vi "Anritsu VNA Set Measurement.vi"(4 "Trace":i8=1 min=1 max=99 step=1, 5 "Parameter":T2={"Stimulus Port"=1, "Response Port"=1} {"Stimulus Port" min=1 step=1; "Response Port" min=1 step=1}, 6 "Channel":i8=1 min=1 max=99 step=1, 7 "Anritsu VNA":T1, 8 "error in (no error)":errorcluster, 11 "VISA Resource Name":refnum<visa-resource-name>) -> (0 "error out":errorcluster, 3 "dup VISA Resource Name":refnum<visa-resource-name>)   [LabVIEW 2011]
doc: "This VI for the HP8753B Network Analyzer sets the measurement."
uses:
  tests/S Parameter/TypeDefs/SP Parameter.ctl
  TypeDefs/Anritsu VNA Instrument Info.ctl
  TypeDefs/Anritsu VNA MS2024A and MS2026A Measurement.ctl
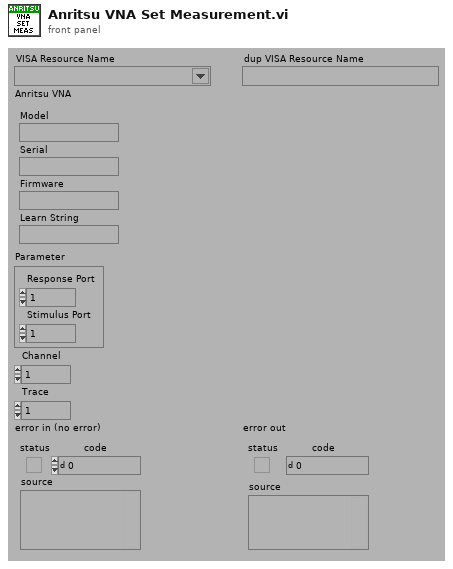
[diagram p1: front panel]
types:
  T1 = typedef "Anritsu VNA Instrument Info.ctl" = cluster{"Model":string, "Serial":string, "Firmware":string, "Learn String":string}
  T2 = typedef "SP Parameter.ctl" = cluster{"Stimulus Port":i8, "Response Port":i8}
  T3 = typedef "Anritsu VNA Model.ctl" = enum16{"Not Supported", "37XXXX", "MS20XXX", "MS462XX", "MS464XX"}
  T4 = typedef "Anritsu VNA MS2024A and MS2026A Measurement.ctl" = enum32{"S11 - Group Delay", "S11 - Log Mag Fault Location", "S11 - Log Mag", "S11 - Phase", "S11 - Smith", "S11 - VSWR Fault Location", "S11 - VSWR", "S21 - Group Delay", "S21 - Log Mag", "S21 - Phase"}
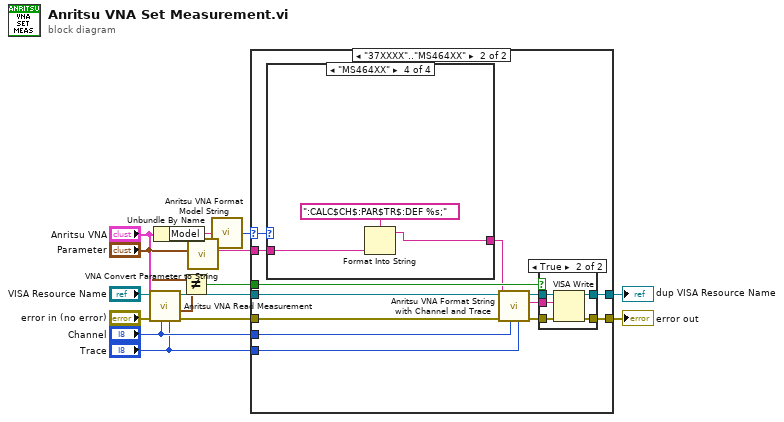
[diagram p0: block diagram]
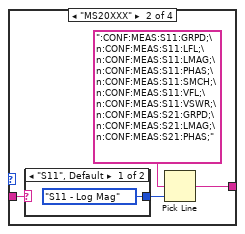
[diagram p5: hidden frame]
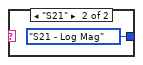
[diagram p6: hidden frame]
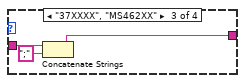
[diagram p7: hidden frame]
diagram:
  n1 = call "Anritsu VNA Read Measurement.vi"("Trace"="Trace", "Channel"="Channel", "Anritsu VNA"="Anritsu VNA", "error in (no error)"="error in (no error)", "VISA Resource Name"="VISA Resource Name") -> ("error out"=w10:errorcluster, "Parameter"=w3:T2, "dup VISA Resource Name"=w9:refnum<visa-resource-name>)  [unwired: 1 in, 3 out]
  n2 = Unbundle By Name("Anritsu VNA") -> ("Model"=w5:string)
  n3 = Not Equal?(x="Parameter", y=w3) -> (x != y?=w7:bool)
  n4 = call "VNA Convert Parameter to String.vi"("Parameter"="Parameter") -> ("Parameter String"=w13:string)  [unwired: 10 out]
  n5 = call "Anritsu VNA Format Model String.vi"("Model"=w5) -> ("Model"=w4:T3)
  n6 = case shown="\"37XXXX\"..\"MS464XX\"" w4 {
    selector: w4 -> [_ w22]
    tunnel: [w17 w28] -> w15
    tunnel: [w16 w27] -> w14
    tunnel: w13 -> [_ w26]
    tunnel: w10 -> [w16 w25]
    tunnel: w9 -> [w17 w24]
    tunnel: w7 -> [_ w23]
    tunnel: "Trace" -> [_ w19]
    tunnel: "Channel" -> [_ w18]
    frame "Not Supported" {
    }
    frame "37XXXX".."MS464XX" {
      n7 = case shown="\"MS464XX\"" w22 {
        tunnel: [_ w38 w44 w45] -> w20
        tunnel: w26 -> [_ w37 w42 w46]
        frame "Not Supported" {
        }
        frame "MS20XXX" {
          n8 = case shown="\"S11\", Default" w37 {
            tunnel: [Anritsu_VNA_MS2024A_and_MS2026A_Measurement."S11 - Log Mag" ("Measurement (S11 - Log Mag)") Anritsu_VNA_MS2024A_and_MS2026A_Measurement."S21 - Log Mag" ("Measurement (S11 - Log Mag)")] -> w36
            frame "S11", Default {
            }
            frame "S21" {
            }
          }
          n9 = Pick Line(multi-line string=":CONF:MEAS:S11:GRPD;\n:CONF:MEAS:S11:LFL;\n:CONF:MEAS:S11:LMAG;\n:CONF:MEAS:S11:PHAS;\n:CONF:MEAS:S11:SMCH;\n:CONF:MEAS:S11:VFL;\n:CONF:MEAS:S11:VSWR;\n:CONF:MEAS:S21:GRPD;\n:CONF:MEAS:S21:LMAG;\n:CONF:MEAS:S21:PHAS;", line index=w36) -> (output string=w38:string)  [unwired: 1 out]
        }
        frame "37XXXX", "MS462XX" {
          n10 = Concatenate Strings(w42, ";" ("string")) -> (w44:string)
        }
        frame "MS464XX" {
          n11 = Format Into String(format string=":CALC$CH$:PAR$TR$:DEF %s;" ("string"), w46) -> (resulting string=w45:string)  [unwired: 2 in, 1 out]
        }
      }
      n12 = call "Anritsu VNA Format String with Channel and Trace.vi"("Trace"=w19, "Channel"=w18, "String"=w20) -> ("String Out"=w21:string)  [unwired: 6 out]
      n13 = case shown="True" w23 {
        tunnel: w21 -> [_ w35]
        tunnel: [w30 w34] -> w28
        tunnel: [w29 w33] -> w27
        tunnel: w25 -> [w29 w32]
        tunnel: w24 -> [w30 w31]
        frame False {
        }
        frame True {
          n14 = VISA Write(VISA resource name=w31, write buffer=w35, error in (no error)=w32) -> (VISA resource name out=w34:refnum<visa-resource-name>, error out=w33:errorcluster)  [unwired: 1 out]
        }
      }
    }
  }
  "dup VISA Resource Name" <- w15
  "error out" <- w14
